vi "DUAL GAUGE-Get Programnumber.vi"(8 "Fehler (Eingang)":errorcluster, 11 "Referenz in":refnum<visa-resource-name>) -> (0 "Cluster (Ausgang)":errorcluster, 1 "Programversion":string, 3 "Referenz out":refnum<visa-resource-name>)   [LabVIEW 2010, in "Dual Gauge.lvlib"]
uses:
  Dual Gauge.lvlib
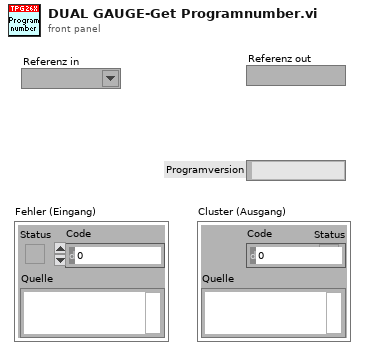
[diagram p1: front panel]
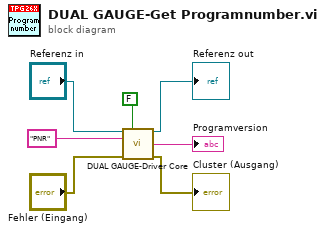
[diagram p0: block diagram]
diagram:
  n1 = call "DUAL GAUGE-Driver Core.vi"("Referenz in"="Referenz in", "Write/Read"=FALSE, "Command"="PNR", "Fehler (Eingang)"="Fehler (Eingang)") -> ("Referenz out"=→"Referenz out":refnum<visa-resource-name>, "String Out"=→"Programversion":string, "Cluster (Ausgang)"=→"Cluster (Ausgang)":errorcluster)  [unwired: 9 in]
